vi "snap.vi"(0 "HGF_IMAQDevice":refnum<class "HGF_IMAQDevice.lvclass">, 2 "Image In":T1, 5 "error in (no error)":errorcluster, 6 "Region of Interest":i32[](array[numeric]), 7 "Step x":i32=-1, 8 "Channel":i32=-1, 9 "Step y":i32=-1) -> (14 "dup HGF_IMAQDevice":refnum<class "HGF_IMAQDevice.lvclass">, 16 "Image Out":T1, 19 "error out":errorcluster)   [LabVIEW 2014, in "HGF_IMAQ.lvlib" / "HGF_IMAQDevice.lvclass"]
doc: "Acquires a single image into <B>Image out</B>. A snap is appropriate for low-speed or single-capture applications where ease of programming is essential.\n\nParameter, except Image, are used for framegrabber, only, and can be ignored for IMAQdx and IMAQ for USB."
uses:
  HGF_IMAQDevice.lvclass
  <vilib>/vision/Image Controls.llb/IMAQ Image.ctl
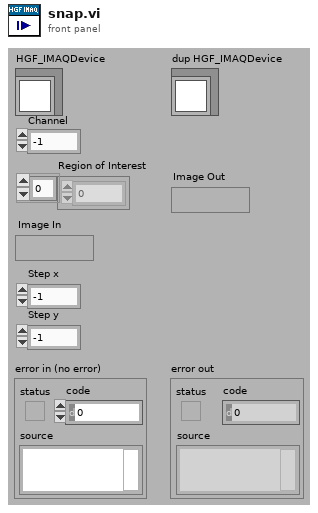
[diagram p1: front panel]
types:
  T1 = typedef "IMAQ Image.ctl" = refnum<image>
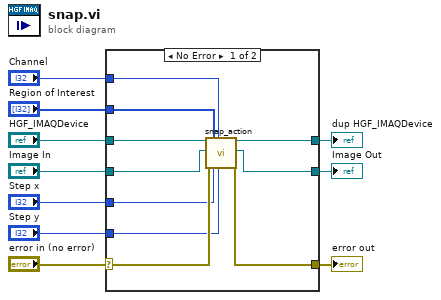
[diagram p0: block diagram]
diagram:
  n1 = case shown="No Error" "error in (no error)" {
    selector: "error in (no error)" -> [w18 w23]
    tunnel: [w17 w23] -> w9
    tunnel: [w19 w22] -> w7
    tunnel: "HGF_IMAQDevice" -> [w20 w22]
    tunnel: [w15 w21] -> w6
    tunnel: "Image In" -> [w16 w21]
    tunnel: "Region of Interest" -> [w14 _]
    tunnel: "Channel" -> [w13 _]
    tunnel: "Step x" -> [w12 _]
    tunnel: "Step y" -> [w11 _]
    frame No Error {
      n2 = call-dynamic "snap_action.vi"("HGF_IMAQDevice"=w20, "Image In"=w16, "error in (no error)"=w18, "Region of Interest"=w14, "Step x"=w12, "Channel"=w13, "Step y"=w11) -> ("dup HGF_IMAQDevice"=w19:refnum<class "HGF_IMAQDevice.lvclass">, "Image Out"=w15:T1, "error out"=w17:errorcluster)  [unwired: 10 out]
    }
    frame Error {
    }
  }
  "error out" <- w9
  "dup HGF_IMAQDevice" <- w7
  "Image Out" <- w6
